vi "AddTextToFile.vi"(8 "Ajouter du texte":string, 11 "Fichier":path) -> ()   [LabVIEW 2022 SP3]
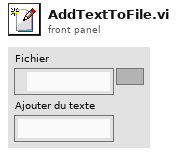
[diagram p1: front panel]
types:
  T1 = enum16{"open", "replace", "create", "open or create", "replace or create", "replace or create with confirmation"}
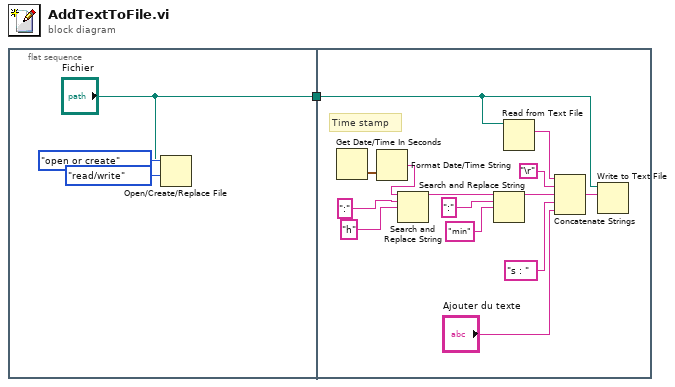
[diagram p0: block diagram]
diagram:
  n1 = flat-sequence {
    tunnel: ["Fichier"] -> w1
    tunnel: w1 -> [w7]
    frame #0 {
      n2 = Open/Create/Replace File(file path (use dialog)="Fichier", operation (0:open)=T1."open or create", access (0:read/write)=enum16{"read/write", "read-only", "write-only"}."read/write") -> ()  [unwired: 3 in, 3 out]
    }
    frame #1 {
      # "Time stamp"
      n3 = Get Date/Time In Seconds() -> (seconds since 1Jan1904=w18:timestamp)
      n4 = Format Date/Time String(seconds (now)=w18) -> (date/time string=w10:string)  [unwired: 2 in]
      n5 = Search and Replace String(input string=w10, search string=":", replace string="h") -> (result string=w15:string)  [unwired: 5 in, 3 out]
      n6 = Search and Replace String(input string=w15, search string=":", replace string="min" ("replace string (\"\")")) -> (result string=w16:string)  [unwired: 5 in, 3 out]
      n7 = Read from Text File(file (use dialog)=w7) -> (text=w14:string)  [unwired: 3 in, 3 out]
      n8 = Concatenate Strings(w14, "\r", w16, "s : ", "Ajouter du texte") -> (w13:string)
      n9 = Write to Text File(file (use dialog)=w7, text=w13) -> ()  [unwired: 2 in, 3 out]
    }
  }
